vi "Main.vi"() -> ()   [LabVIEW 2015]
doc: "The myRIO Project template acquires acceleration data from the onboard accelerometer and displays the changes of acceleration values in a waveform chart."
uses:
  <vilib>/myRIO/Instrument Drivers/Onboard IO/PWM/typedefs/PWM Reference.ctl
  <vilib>/myRIO/Common/Instrument Driver Framework/Utilities/typedefs/myRIO Generic Hardware Reference.ctl
  <vilib>/myRIO/Common/Instrument Driver Framework/Utilities/typedefs/Hardware Version Enum.ctl
  <vilib>/myRIO/Common/Instrument Driver Framework/Utilities/typedefs/myRIO v1.0 Reference.ctl
  <vilib>/myRIO/Common/Instrument Driver Framework/Utilities/typedefs/Generic FPGA Reference.ctl
  <vilib>/myRIO/Common/Instrument Driver Framework/myRIO v1.0/PWM/typedefs/PWM Channels Enum.ctl
  <vilib>/myRIO/Instrument Drivers/Onboard IO/PWM/typedefs/PWM Configuration.ctl
  <vilib>/userdefined/High Color/nirio_resource_hc.ctl
  <vilib>/myRIO/Instrument Drivers/Onboard IO/DIO/typedefs/DIO Reference.ctl
  <vilib>/myRIO/Common/Instrument Driver Framework/myRIO v1.0/DIO/typedefs/DIO Channels List.ctl
  <vilib>/myRIO/Common/Instrument Driver Framework/myRIO v1.0/DIO/typedefs/DIO Channels Enum.ctl
  <vilib>/myRIO/Instrument Drivers/Onboard IO/AI/typedefs/AI Reference.ctl
  <vilib>/myRIO/Common/Instrument Driver Framework/myRIO v1.0/AI/typedefs/AI Channels List.ctl
  <vilib>/myRIO/Common/Instrument Driver Framework/myRIO v1.0/AI/typedefs/AI Channels Enum.ctl
  <vilib>/myRIO/Common/Instrument Driver Framework/Utilities/typedefs/Analog Scaling Constants List.ctl
  <vilib>/myRIO/Common/Instrument Driver Framework/Utilities/typedefs/Analog Scaling Constants.ctl
  <vilib>/myRIO/Instrument Drivers/Onboard Devices/Accelerometer/typedefs/Accelerometer Reference.ctl
  <vilib>/myRIO/Common/Instrument Driver Framework/myRIO v1.0/Accelerometer/typedefs/Accelerometer Channels List.ctl
  <vilib>/myRIO/Common/Instrument Driver Framework/myRIO v1.0/Accelerometer/typedefs/Accelerometer Channels Enum.ctl
  <vilib>/myRIO/Common/Instrument Driver Framework/Utilities/vis/Is FPGA Ref Available.vi
  <vilib>/myRIO/Common/Instrument Driver Framework/myRIO v1.0/DIO/vis/myRIO v1.1 Open DIO.vi
  <vilib>/myRIO/Instrument Drivers/Onboard IO/DIO/vis/Read.vi
  <vilib>/myRIO/Common/Instrument Driver Framework/myRIO v1.0/AI/vis/myRIO v1.1 Open AI.vi
  <vilib>/myRIO/Instrument Drivers/Onboard IO/AI/vis/Read.vi
  <vilib>/myRIO/Instrument Drivers/Onboard IO/DIO/vis/Write.vi
  <vilib>/myRIO/Common/Instrument Driver Framework/myRIO v1.0/PWM/vis/myRIO v1.1 Open PWM.vi
  <vilib>/myRIO/Instrument Drivers/Onboard IO/PWM/vis/Set Duty Cycle and Frequency.vi
  <vilib>/myRIO/Common/Instrument Driver Framework/myRIO v1.0/Accelerometer/vis/myRIO v1.1 Open Accelerometer.vi
  <vilib>/myRIO/Instrument Drivers/Onboard Devices/Accelerometer/vis/Read.vi
  <vilib>/myRIO/Common/Instrument Driver Framework/Utilities/vis/Validate Channels.vi
  <vilib>/myRIO/Common/Instrument Driver Framework/myRIO v1.0/DIO/vis/myRIO v1.0 Reserve DIO.vi
  <vilib>/myRIO/Common/Instrument Driver Framework/myRIO v1.0/AI/vis/myRIO v1.0 Reserve AI.vi
  <vilib>/myRIO/Common/Instrument Driver Framework/myRIO v1.0/PWM/vis/myRIO v1.0 Reserve PWM.vi
  <vilib>/myRIO/Common/Instrument Driver Framework/myRIO v1.0/Accelerometer/vis/myRIO v1.0 Reserve Accelerometer.vi
  <vilib>/myRIO/Common/Instrument Driver Framework/myRIO v1.0/UART/vis/myRIO v1.0 Close UART.vi
  <vilib>/myRIO/Common/Instrument Driver Framework/myRIO v1.0/Resource Manager/vis/myRIO v1.0 Reserve Channel List.vi
  <vilib>/myRIO/Common/Instrument Driver Framework/myRIO v1.0/DIO/vis/myRIO v1.0 Build MUX Configuration DIO.vi
  <vilib>/myRIO/Common/Instrument Driver Framework/myRIO v1.0/AI/vis/myRIO v1.0 Build MUX Configuration AI.vi
  <vilib>/myRIO/Common/Instrument Driver Framework/myRIO v1.0/PWM/vis/myRIO v1.0 Build MUX Configuration PWM.vi
  <vilib>/myRIO/Common/Instrument Driver Framework/myRIO v1.0/Accelerometer/vis/myRIO v1.0 Build MUX Configuration Accelerometer.vi
  <vilib>/myRIO/Common/Instrument Driver Framework/myRIO v1.0/Resource Manager/vis/myRIO v1.0 Reserve Channel.vi
  <vilib>/myRIO/Common/Instrument Driver Framework/myRIO v1.0/Resource Manager/vis/myRIO v1.0 Unreserve Channel.vi
  <vilib>/myRIO/Common/Instrument Driver Framework/myRIO v1.0/Resource Manager/vis/myRIO v1.0 Create Configuration List.vi
  <vilib>/myRIO/Common/Instrument Driver Framework/myRIO v1.0/Resource Manager/vis/myRIO v1.0 Build Mutex Name.vi
  <vilib>/Utility/VariantDataType/GetNumericInfo.vi
  <vilib>/Utility/error.llb/Error Cluster From Error Code.vi
  <vilib>/myRIO/Common/Instrument Driver Framework/myRIO v1.0/myRIO v1.1 Open.vi
  <vilib>/myRIO/Common/Instrument Driver Framework/Utilities/vis/IO Manager.vi
  <vilib>/myRIO/Common/Instrument Driver Framework/Utilities/vis/Configuration Manager.vi
  <vilib>/myRIO/Common/Instrument Driver Framework/myRIO v1.0/Resource Manager/vis/myRIO v1.0 Configure IO.vi
  <vilib>/myRIO/Common/Instrument Driver Framework/myRIO v1.0/myRIO v1.0 Close.vi
  <vilib>/myRIO/Common/Instrument Driver Framework/myRIO v1.0/PWM/vis/myRIO v1.0 Write PWM.vi
  <vilib>/myRIO/Common/Instrument Driver Framework/myRIO v1.0/DIO/vis/myRIO v1.0 Read DIO.vi
  <vilib>/myRIO/Common/Instrument Driver Framework/myRIO v1.0/AI/vis/myRIO v1.0 Get Scaling Constants AI.vi
  <vilib>/myRIO/Common/Instrument Driver Framework/myRIO v1.0/AI/vis/myRIO v1.0 Read AI.vi
  <vilib>/myRIO/Common/Instrument Driver Framework/myRIO v1.0/DIO/vis/myRIO v1.0 Write DIO.vi
  <vilib>/myRIO/Common/Instrument Driver Framework/myRIO v1.0/Accelerometer/vis/myRIO v1.0 Get Scaling Constant Accelerometer.vi
  <vilib>/myRIO/Common/Instrument Driver Framework/myRIO v1.0/Accelerometer/vis/myRIO v1.0 Read Accelerometer.vi
  <vilib>/myRIO/Common/Instrument Driver Framework/Utilities/vis/FPGA Ref Manager.vi
  <vilib>/myRIO/Common/Instrument Driver Framework/myRIO v1.0/myRIO v1.0 Reset FPGA.vi
  <vilib>/myRIO/Common/Instrument Driver Framework/myRIO v1.0/IRQ/vis/myRIO v1.0 IRQ Info FGV.vi
  <vilib>/myRIO/Common/Instrument Driver Framework/myRIO v1.0/IRQ/vis/myRIO v1.0 Timer IRQ Info FGV.vi
  <vilib>/myRIO/Common/Instrument Driver Framework/myRIO v1.0/IRQ/vis/myRIO v1.0 ISR Agent.vi
  <vilib>/myRIO/Express VI/Onboard IO/PWM/PWM Express VI.xnode
  <vilib>/myRIO/Instrument Drivers/Onboard IO/PWM/vis/myRIO PWM Open.xnode
  <vilib>/myRIO/Express VI/Onboard IO/DI/DI Express VI.xnode
  <vilib>/myRIO/Instrument Drivers/Onboard IO/DIO/vis/myRIO DIO Open.xnode
  <vilib>/myRIO/Express VI/Onboard IO/AI/AI Express VI.xnode
  <vilib>/myRIO/Instrument Drivers/Onboard IO/AI/vis/myRIO AI Open.xnode
  <vilib>/myRIO/Express VI/Onboard IO/DO/DO Express VI.xnode
  <vilib>/myRIO/Express VI/Onboard Devices/Accelerometer/Accelerometer Express VI.xnode
  <vilib>/myRIO/Instrument Drivers/Onboard Devices/Accelerometer/vis/myRIO Accelerometer Open.xnode
  <vilib>/myRIO/Instrument Drivers/Utilities/Utilities.lvlib
  <vilib>/myRIO/Instrument Drivers/Onboard Devices/Accelerometer/Accelerometer.lvlib
  <vilib>/myRIO/Instrument Drivers/Onboard IO/PWM/PWM.lvlib
  <vilib>/myRIO/Instrument Drivers/Onboard IO/DIO/DIO.lvlib
  <vilib>/myRIO/Instrument Drivers/Onboard IO/AI/AI.lvlib
panel:
  in  "Frequency [Hz] 2":dbl=40000.0
  in  "Duty Cycle":dbl=0.01
  in  "旋钮":dbl(knob) scale=0.025..0.125
  in  "Frequency [Hz]":dbl=1000.0
  out "B/DIO0 (Pin 11)":bool
  out "A/DIO0 (Pin 11)":bool
  out "A/AI1 (Pin 5)":dbl
  out "A/AI0 (Pin 3)":dbl
  out "结果":dbl
  out "X-Axis":dbl
  out "波形图表":T1(graph)
  out "error out":errorcluster
  # "Overview: The myRIO Project template acquires acceleration data from the onboard accelerometer and displays the changes of acceleration values in a waveform chart.\nInstructions:\n1. Check the myRIO target IP address in the project and make sure the target IP address is correct. \n2. Run this VI."
  # "左 29"
  # "右31"
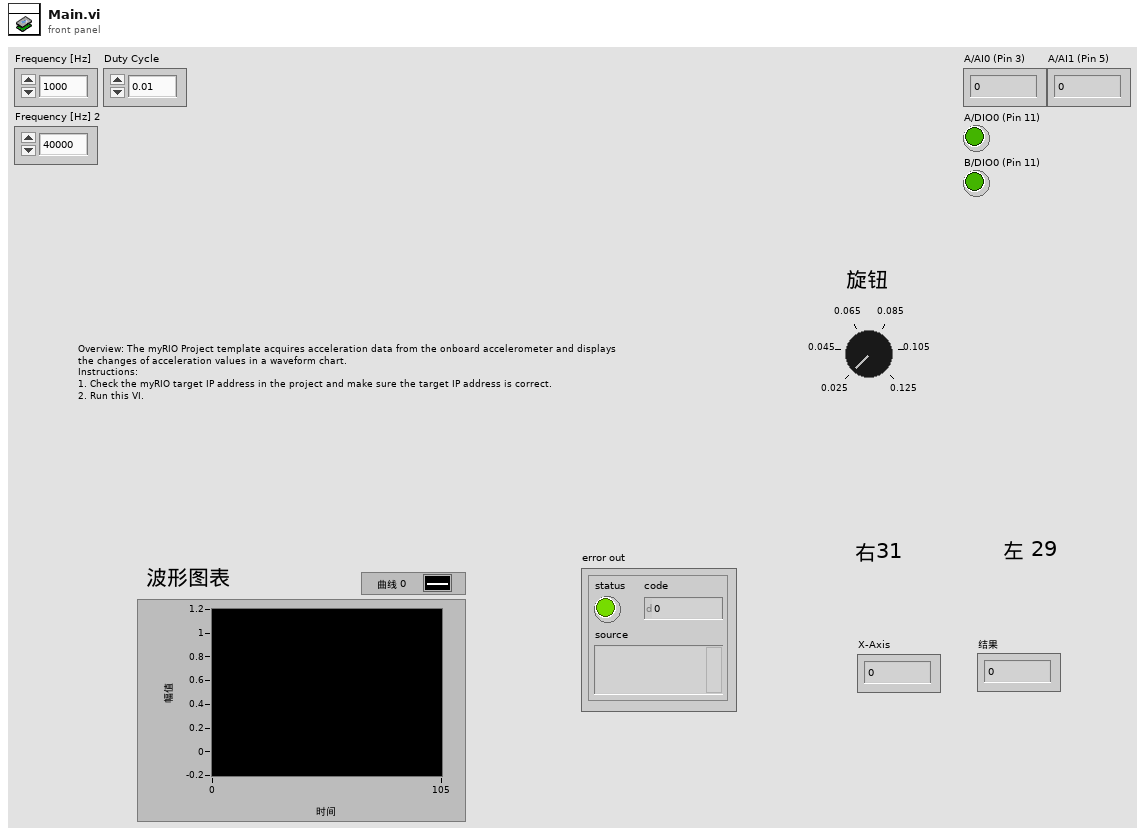
[diagram p1: front panel]
types:
  T1 = cluster{"X-Axis":dbl, "Y-Axis":dbl, "Z-Axis":dbl}
  T2 = typedef "DIO.lvlib/DIO Reference.ctl" = cluster{"myRIO Reference":T3, "DIO Channels List":T7}
  T3 = typedef "myRIO Generic Hardware Reference.ctl" = cluster{"myRIO Model":T4, "myRIO Hardware Reference":T5}
  T4 = typedef "Hardware Version Enum.ctl" = enum16{"Unknown", "myRIO-1900", "myRIO-1950", "roboRIO"}
  T5 = typedef "myRIO v1.0 Reference.ctl" = cluster{"Generic FPGA Reference":T6, "Allow multiple opens":bool}
  T6 = typedef "Generic FPGA Reference.ctl" = refnum<k20>
  T7 = typedef "DIO Channels List.ctl" = T8[]
  T8 = typedef "DIO Channels Enum.ctl" = enum16{"Not Connected", "C/DIO0", "C/DIO1", "C/DIO2", "C/DIO3", "C/DIO4", "C/DIO5", "C/DIO6", "C/DIO7", "A/DIO0", "A/DIO1", "A/DIO2", "A/DIO3", "A/DIO4", "A/DIO5", "A/DIO6", "A/DIO7", "A/DIO8", "A/DIO9", "A/DIO10", "A/DIO11", "A/DIO12", "A/DIO13", "A/DIO14", "A/DIO15", "B/DIO0", "B/DIO1", "B/DIO2", "B/DIO3", "B/DIO4", "B/DIO5", "B/DIO6", "B/DIO7", "B/DIO8", "B/DIO9", "B/DIO10", "B/DIO11", "B/DIO12", "B/DIO13", "B/DIO14", "B/DIO15", "LED0", "LED1", "LED2", "LED3", "Button0", "DIO/DIO0", "DIO/DIO1", "DIO/DIO2", "DIO/DIO3", "DIO/DIO4", "DIO/DIO5", "DIO/DIO6", "DIO/DIO7", "DIO/DIO8", "DIO/DIO9", "SPI/CS0", "SPI/CS1", "SPI/CS2", "SPI/CS3", "LED RADIO (Green)", "LED RADIO (Red)", "LED COMM (Green)", "LED COMM (Red)", "LED MODE (Green)", "LED MODE (Red)"}
  T9 = typedef "nirio_resource_hc.ctl" = tag
  T10 = typedef "PWM.lvlib/PWM Reference.ctl" = cluster{"myRIO Reference":T3, "PWM Channels Enum":T11, "PWM Configuration":T12}
  T11 = typedef "PWM Channels Enum.ctl" = enum16{"Not Connected", "C/PWM0", "C/PWM1", "A/PWM0", "A/PWM1", "A/PWM2", "B/PWM0", "B/PWM1", "B/PWM2", "PWM/PWM0", "PWM/PWM1", "PWM/PWM2", "PWM/PWM3", "PWM/PWM4", "PWM/PWM5", "PWM/PWM6", "PWM/PWM7", "PWM/PWM8", "PWM/PWM9"}
  T12 = typedef "PWM.lvlib/PWM Configuration.ctl" = cluster{"Frequency":dbl, "Duty Cycle":dbl}
  T13 = typedef "AI.lvlib/AI Reference.ctl" = cluster{"myRIO Reference":T3, "AI Channels List":T14, "AI Scaling Constants List":T16}
  T14 = typedef "AI Channels List.ctl" = T15[]
  T15 = typedef "AI Channels Enum.ctl" = enum16{"Not Connected", "AudioIn/Left", "AudioIn/Right", "C/AI0", "C/AI1", "A/AI0", "A/AI1", "A/AI2", "A/AI3", "B/AI0", "B/AI1", "B/AI2", "B/AI3", "AI/AI0", "AI/AI1", "AI/AI2", "AI/AI3"}
  T16 = typedef "Analog Scaling Constants List.ctl" = T17[]
  T17 = typedef "Analog Scaling Constants.ctl" = cluster{"LSB Weight (Volts)":dbl, "Offset (Volts)":dbl, "Signed?":bool}
  T18 = typedef "Accelerometer.lvlib/Accelerometer Reference.ctl" = cluster{"myRIO Reference":T3, "Accelerometer Channels List":T19, "LSB Weight":dbl}
  T19 = typedef "Accelerometer Channels List.ctl" = T20[]
  T20 = typedef "Accelerometer Channels Enum.ctl" = enum16{"Not Connected", "X-Axis", "Y-Axis", "Z-Axis"}
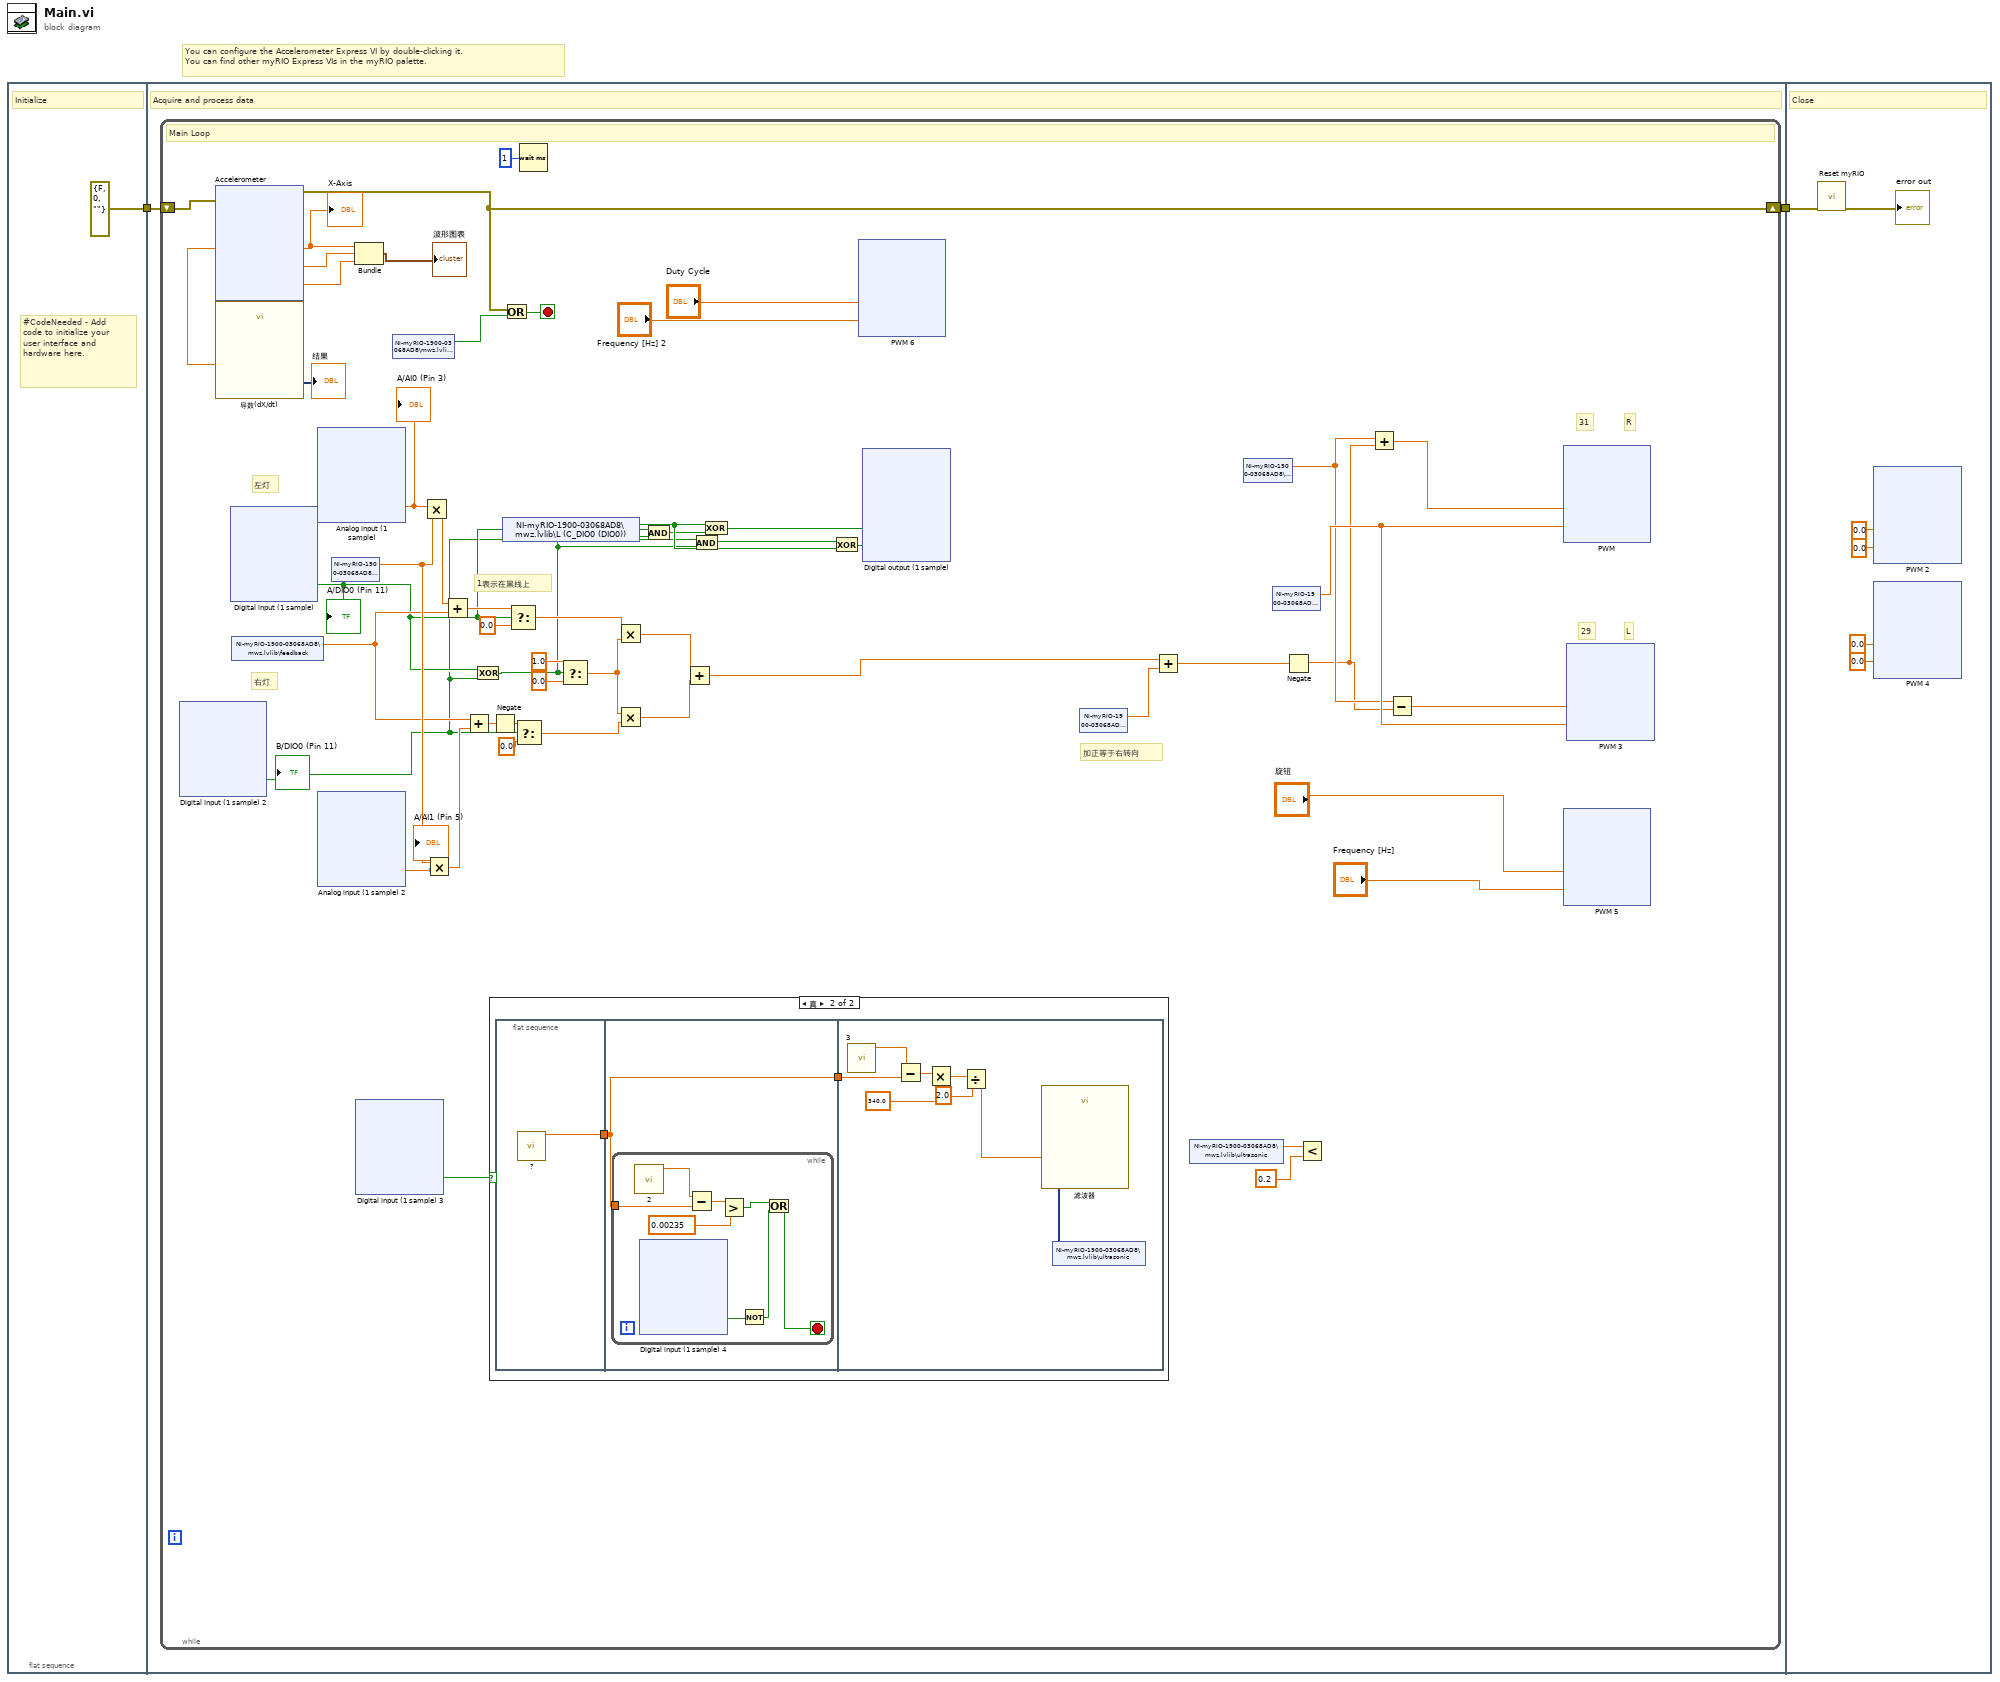
[diagram p0: block diagram]
diagram:
  # "You can configure the Accelerometer Express VI by double-clicking it.\nYou can find other myRIO Express VIs in the myRIO palette."
  n1 = flat-sequence {
    tunnel: [errorcluster {"status"=FALSE, "code"=0, "source"=""} ("error in (no error)")] -> w2
    tunnel: w2 -> [w5]
    tunnel: [w4] -> w1
    tunnel: w1 -> [w511]
    frame #0 {
      # "#CodeNeeded - Add code to initialize your user interface and hardware here."
      # "Initialize"
    }
    frame #1 {
      # "Acquire and process data"
      n2 = while {
        shift-right: [w54] -> w4
        shift-left: w5 -> [w23]
        stop <- w56 stop-if-true
        # "L"
        # "R"
        # "加正等于右转向"
        # "1表示在黑线上"
        # "右灯"
        # "左灯"
        # "29"
        # "31"
        # "Main Loop"
        n3 = xnode "Digital input (1 sample) 2"() -> ("B/DIO0 (Pin 11)"=w14:bool)  [unwired: 1 in, 1 out]
        "B/DIO0 (Pin 11)" <- w14
        n4 = xnode "Accelerometer"("error in (no error)"=w23) -> ("X-Axis"=w22:dbl, "Y-Axis"=w53:dbl, "Z-Axis"=w52:dbl, "error out"=w54:errorcluster)
        "X-Axis" <- w22
        n5 = call "导数(dX/dt)"("Signals"=w22) -> ("Result"=→"结果":dynamicdata)  [unwired: 5 in, 1 out]
        n6 = xnode "Digital input (1 sample)"() -> ("A/DIO0 (Pin 11)"=w16:bool)  [unwired: 1 in, 1 out]
        "A/DIO0 (Pin 11)" <- w16
        n7 = shared-variable "NI-myRIO-1900-03068AD8\\mwz.lvlib\\feedback"() -> (w24:dbl)  [unwired: 1 in, 1 out]
        n8 = xnode "Analog input (1 sample)"() -> ("A/AI0 (Pin 3)"=w31:dbl)  [unwired: 1 in, 1 out]
        "A/AI0 (Pin 3)" <- w31
        n9 = xnode "Analog input (1 sample) 2"() -> ("A/AI1 (Pin 5)"=w28:dbl)  [unwired: 1 in, 1 out]
        "A/AI1 (Pin 5)" <- w28
        n10 = shared-variable "NI-myRIO-1900-03068AD8\\mwz.lvlib\\a"() -> (w27:dbl)  [unwired: 1 in, 1 out]
        n11 = Bundle("X-Axis"=w22, "Y-Axis"=w53, "Z-Axis"=w52) -> (→"波形图表":T1)  [unwired: 1 in]
        n12 = xnode "Digital input (1 sample) 3"() -> ("B/DIO15 (Pin 34)"=w8:bool)  [unwired: 1 in, 1 out]
        n13 = shared-variable "NI-myRIO-1900-03068AD8\\mwz.lvlib\\OFF"() -> (w50:bool)  [unwired: 1 in, 1 out]
        n14 = Multiply(x=w31, y=w27) -> (x*y=w29:dbl)
        n15 = Multiply(x=w27, y=w28) -> (x*y=w26:dbl)
        n16 = Add(x=w29, y=w24) -> (x+y=w30:dbl)
        n17 = Add(x=w24, y=w26) -> (x+y=w25:dbl)
        n18 = Exclusive Or(1:w14, 2:w16) -> (0:w13:bool)
        n19 = case shown="真" w8 {
          frame False {
          }
          frame True {
            n20 = flat-sequence {
              tunnel: [w94] -> w93
              tunnel: w93 -> [w95]
              tunnel: [w95] -> w92
              tunnel: w92 -> [w145]
              frame #0 {
                n21 = call "?"() -> ("Present (s)"=w94:dbl)  [unwired: 12 in, 7 out]
              }
              frame #1 {
                n22 = while {
                  tunnel: w95 -> [w102]
                  stop <- w96 stop-if-true
                  n23 = call "2"() -> ("Present (s)"=w103:dbl)  [unwired: 12 in, 7 out]
                  n24 = xnode "Digital input (1 sample) 4"() -> ("B/DIO15 (Pin 34)"=w98:bool)  [unwired: 1 in, 1 out]
                  n25 = Subtract(x=w103, y=w102) -> (x-y=w101:dbl)
                  n26 = Greater?(x=w101, y=0.00235) -> (0:w99:bool)
                  n27 = Not(x=w98) -> (.not. x?=w97:bool)
                  n28 = Or(x=w99, y=w97) -> (x .or. y?=w96:bool)
                }
              }
              frame #2 {
                n29 = call "3"() -> ("Present (s)"=w146:dbl)  [unwired: 12 in, 7 out]
                n30 = Subtract(x=w146, y=w145) -> (x-y=w144:dbl)
                n31 = Multiply(x=w144, y=340.0) -> (x*y=w142:dbl)
                n32 = Divide(x=w142, y=2.0) -> (x/y=w140:dbl)
                n33 = call "滤波器"("Signal"=w140) -> ("Filtered Signal"=w139:dynamicdata)  [unwired: 9 in, 1 out]
                n34 = shared-variable "NI-myRIO-1900-03068AD8\\mwz.lvlib\\ultrasonic"(w139) -> ()  [unwired: 1 in, 1 out]
              }
            }
          }
        }
        n35 = Negate(x=w25) -> (-x=w32:dbl)
        n36 = Or(x=w54, y=w50) -> (x .or. y?=w56:bool)
        n37 = shared-variable "NI-myRIO-1900-03068AD8\\mwz.lvlib\\L (C_DIO0 (DIO0))"() -> (w18:bool)  [unwired: 1 in, 1 out]
        n38 = Select(t=w30, s=w16, f=0.0) -> (s? t:f=w40:dbl)
        n39 = Select(t=w32, s=w14, f=0.0) -> (s? t:f=w39:dbl)
        n40 = Wait (ms)(milliseconds to wait=u32 1) -> ()  [unwired: 1 out]
        n41 = Select(t=1.0, s=w13, f=0.0) -> (s? t:f=w38:dbl)
        n42 = Multiply(x=w40, y=w38) -> (x*y=w37:dbl)
        n43 = Multiply(x=w38, y=w39) -> (x*y=w36:dbl)
        n44 = And(x=w16, y=w13) -> (x .and. y?=w17:bool)
        n45 = Add(x=w37, y=w36) -> (x+y=w34:dbl)
        n46 = And(x=w14, y=w13) -> (x .and. y?=w15:bool)
        n47 = Exclusive Or(1:w17, 2:w18) -> (0:w20:bool)
        n48 = Exclusive Or(1:w18, 2:w15) -> (0:w19:bool)
        n49 = xnode "PWM 6"("Duty Cycle"="Duty Cycle", "Frequency [Hz]"="Frequency [Hz] 2") -> ()  [unwired: 1 in, 1 out]
        n50 = xnode "Digital output (1 sample)"("L (C/DIO0 (DIO0))"=w20, "R (C/DIO1 (DIO1))"=w19) -> ()  [unwired: 1 in, 1 out]
        n51 = shared-variable "NI-myRIO-1900-03068AD8\\mwz.lvlib\\L"() -> (w33:dbl)  [unwired: 1 in, 1 out]
        n52 = Add(x=w34, y=w33) -> (x+y=w35:dbl)
        n53 = shared-variable "NI-myRIO-1900-03068AD8\\mwz.lvlib\\ultrasonic"() -> (w7:dbl)  [unwired: 1 in, 1 out]
        n54 = shared-variable "NI-myRIO-1900-03068AD8\\mwz.lvlib\\R"() -> (w46:dbl)  [unwired: 1 in, 1 out]
        n55 = shared-variable "NI-myRIO-1900-03068AD8\\mwz.lvlib\\F"() -> (w49:dbl)  [unwired: 1 in, 1 out]
        n56 = Negate(x=w35) -> (-x=w45:dbl)
        n57 = Less?(x=w7, y=0.2) -> ()  [unwired: 1 out]
        n58 = Add(x=w46, y=w45) -> (x+y=w47:dbl)
        n59 = Subtract(x=w46, y=w45) -> (x-y=w48:dbl)
        n60 = xnode "PWM"("Duty Cycle"=w47, "Frequency [Hz]"=w49) -> ()  [unwired: 1 in, 1 out]
        n61 = xnode "PWM 5"("Duty Cycle"="旋钮", "Frequency [Hz]"="Frequency [Hz]") -> ()  [unwired: 1 in, 1 out]
        n62 = xnode "PWM 3"("Duty Cycle"=w48, "Frequency [Hz]"=w49) -> ()  [unwired: 1 in, 1 out]
      }
    }
    frame #2 {
      # "Close"
      n63 = call <vilib>:"Reset myRIO.vi"("error in (no error)"=w511) -> ("error out"=→"error out":errorcluster)  [unwired: 10 in]
      n64 = xnode "PWM 2"("Duty Cycle"=0.0, "Frequency [Hz]"=0.0) -> ()  [unwired: 1 in, 1 out]
      n65 = xnode "PWM 4"("Duty Cycle"=0.0, "Frequency [Hz]"=0.0) -> ()  [unwired: 1 in, 1 out]
    }
  }
